vi "Ejercicio_09_filtro_EMA_con_while.vi"() -> ()   [LabVIEW 2020]
panel:
  out "appended array":dbl[](array[numeric])
  in  "stop":bool
  in  "Array":dbl[](array[numeric])
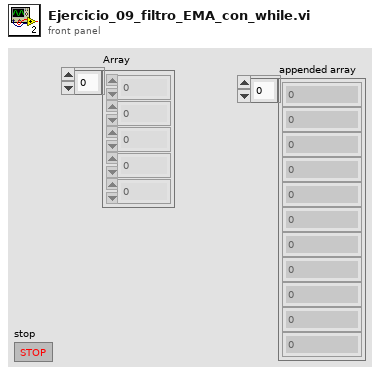
[diagram p1: front panel]
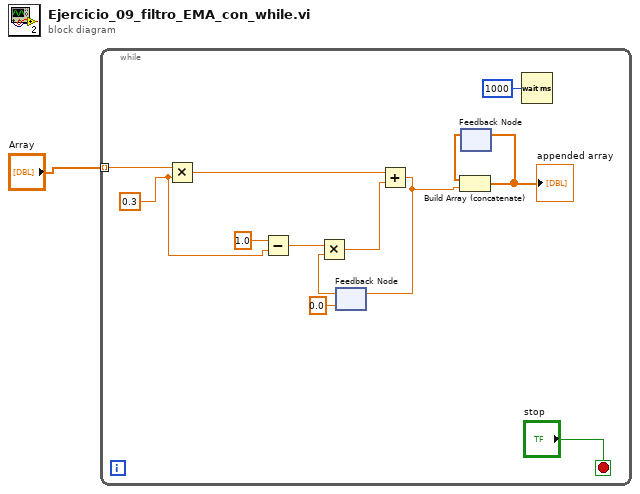
[diagram p0: block diagram]
diagram:
  n1 = while {
    tunnel: "Array" -> [w14] mode=indexing
    stop <- "stop" stop-if-true
    w10 = 0.3 ("y")
    n2 = Multiply(x=w14, y=w10) -> (x*y=w12:dbl)
    n3 = Subtract(x=1.0, y=w10) -> (x-y=w9:dbl)
    n4 = feedback #1(0.0) -> (w7:dbl)
    n5 = Multiply(x=w9, y=w7) -> (x*y=w8:dbl)
    n6 = Add(x=w12, y=w8) -> (x+y=w4:dbl)
    n7 = feedback-in #1(w4) -> ()
    n8 = feedback #2() -> (w2:dbl[])  [unwired: 1 in]
    n9 = Build Array (concatenate)(w2, w4) -> (w3:dbl[])
    "appended array" <- w3
    n10 = feedback-in #2(w3) -> ()
    n11 = Wait (ms)(milliseconds to wait=u32 1000) -> ()  [unwired: 1 out]
  }
